vi "ID Finder.vi"(0 "cluster":T3 {"data[0]"."payload" format="%x"; "data[0]"."timestamp" format="%<%.7X\n%x>T"; "data[0]"."type" items=["CAN Data"=0, "CAN Remote"=1, "CAN Bus Error"=2, "CAN 2.0 Data"=8, "CAN FD Data"=16, "CAN FD+BRS Data"=24, "J1939 Data"=192, "Delay"=224, "Log Trigger"=225, "Start Trigger"=226]; "data[0]"."identifier" format="%x"; "data[1]"."payload" format="%x"; "data[1]"."timestamp" format="%<%.7X\n%x>T"; "data[1]"."type" items=["CAN Data"=0, "CAN Remote"=1, "CAN Bus Error"=2, "CAN 2.0 Data"=8, "CAN FD Data"=16, "CAN FD+BRS Data"=24, "J1939 Data"=192, "Delay"=224, "Log Trigger"=225, "Start Trigger"=226]; "data[1]"."identifier" format="%x"; "data[2]"."payload" format="%x"; "data[2]"."timestamp" format="%<%.7X\n%x>T"; "data[2]"."type" items=["CAN Data"=0, "CAN Remote"=1, "CAN Bus Error"=2, "CAN 2.0 Data"=8, "CAN FD Data"=16, "CAN FD+BRS Data"=24, "J1939 Data"=192, "Delay"=224, "Log Trigger"=225, "Start Trigger"=226]; "data[2]"."identifier" format="%x"; "data[3]"."payload" format="%x"; "data[3]"."timestamp" format="%<%.7X\n%x>T"; "data[3]"."type" items=["CAN Data"=0, "CAN Remote"=1, "CAN Bus Error"=2, "CAN 2.0 Data"=8, "CAN FD Data"=16, "CAN FD+BRS Data"=24, "J1939 Data"=192, "Delay"=224, "Log Trigger"=225, "Start Trigger"=226]; "data[3]"."identifier" format="%x"; "data[4]"."payload" format="%x"; "data[4]"."timestamp" format="%<%.7X\n%x>T"; "data[4]"."type" items=["CAN Data"=0, "CAN Remote"=1, "CAN Bus Error"=2, "CAN 2.0 Data"=8, "CAN FD Data"=16, "CAN FD+BRS Data"=24, "J1939 Data"=192, "Delay"=224, "Log Trigger"=225, "Start Trigger"=226]; "data[4]"."identifier" format="%x"; "data[5]"."payload" format="%x"; "data[5]"."timestamp" format="%<%.7X\n%x>T"; "data[5]"."type" items=["CAN Data"=0, "CAN Remote"=1, "CAN Bus Error"=2, "CAN 2.0 Data"=8, "CAN FD Data"=16, "CAN FD+BRS Data"=24, "J1939 Data"=192, "Delay"=224, "Log Trigger"=225, "Start Trigger"=226]; "data[5]"."identifier" format="%x"; "data[6]"."payload" format="%x"; "data[6]"."timestamp" format="%<%.7X\n%x>T"; "data[6]"."type" items=["CAN Data"=0, "CAN Remote"=1, "CAN Bus Error"=2, "CAN 2.0 Data"=8, "CAN FD Data"=16, "CAN FD+BRS Data"=24, "J1939 Data"=192, "Delay"=224, "Log Trigger"=225, "Start Trigger"=226]; "data[6]"."identifier" format="%x"; "data[7]"."payload" format="%x"; "data[7]"."timestamp" format="%<%.7X\n%x>T"; "data[7]"."type" items=["CAN Data"=0, "CAN Remote"=1, "CAN Bus Error"=2, "CAN 2.0 Data"=8, "CAN FD Data"=16, "CAN FD+BRS Data"=24, "J1939 Data"=192, "Delay"=224, "Log Trigger"=225, "Start Trigger"=226]; "data[7]"."identifier" format="%x"; "data[8]"."payload" format="%x"; "data[8]"."timestamp" format="%<%.7X\n%x>T"; "data[8]"."type" items=["CAN Data"=0, "CAN Remote"=1, "CAN Bus Error"=2, "CAN 2.0 Data"=8, "CAN FD Data"=16, "CAN FD+BRS Data"=24, "J1939 Data"=192, "Delay"=224, "Log Trigger"=225, "Start Trigger"=226]; "data[8]"."identifier" format="%x"}, 1 "ID ESPERADO STRING":string) -> (2 "Identifier":u32 format="%x", 3 "Data Type":T1 items=["CAN Data"=0, "CAN Remote"=1, "CAN Bus Error"=2, "CAN 2.0 Data"=8, "CAN FD Data"=16, "CAN FD+BRS Data"=24, "J1939 Data"=192, "Delay"=224, "Log Trigger"=225, "Start Trigger"=226], 4 "Timestamp":timestamp, 5 "Payload":u8[](array[numeric]) format="%x", 6 "ID String":string, 7 "Data String":string)   [LabVIEW 2023]
uses:
  <vilib>/xnet/xnet.llb/XNET Frame CAN.ctl
  <vilib>/xnet/xnet.llb/XNET Frame Type CAN.ctl
  C:/Elatch-Bench-Test/VIs 64 bits/Users/k90011005/Desktop/Practicas/C#/String-Hexa/bin/Debug/String-Hexa.dll
  VIs 64 bits/Users/k90011005/Desktop/Practicas/C#/String-Hexa/bin/Debug/String-Hexa.dll
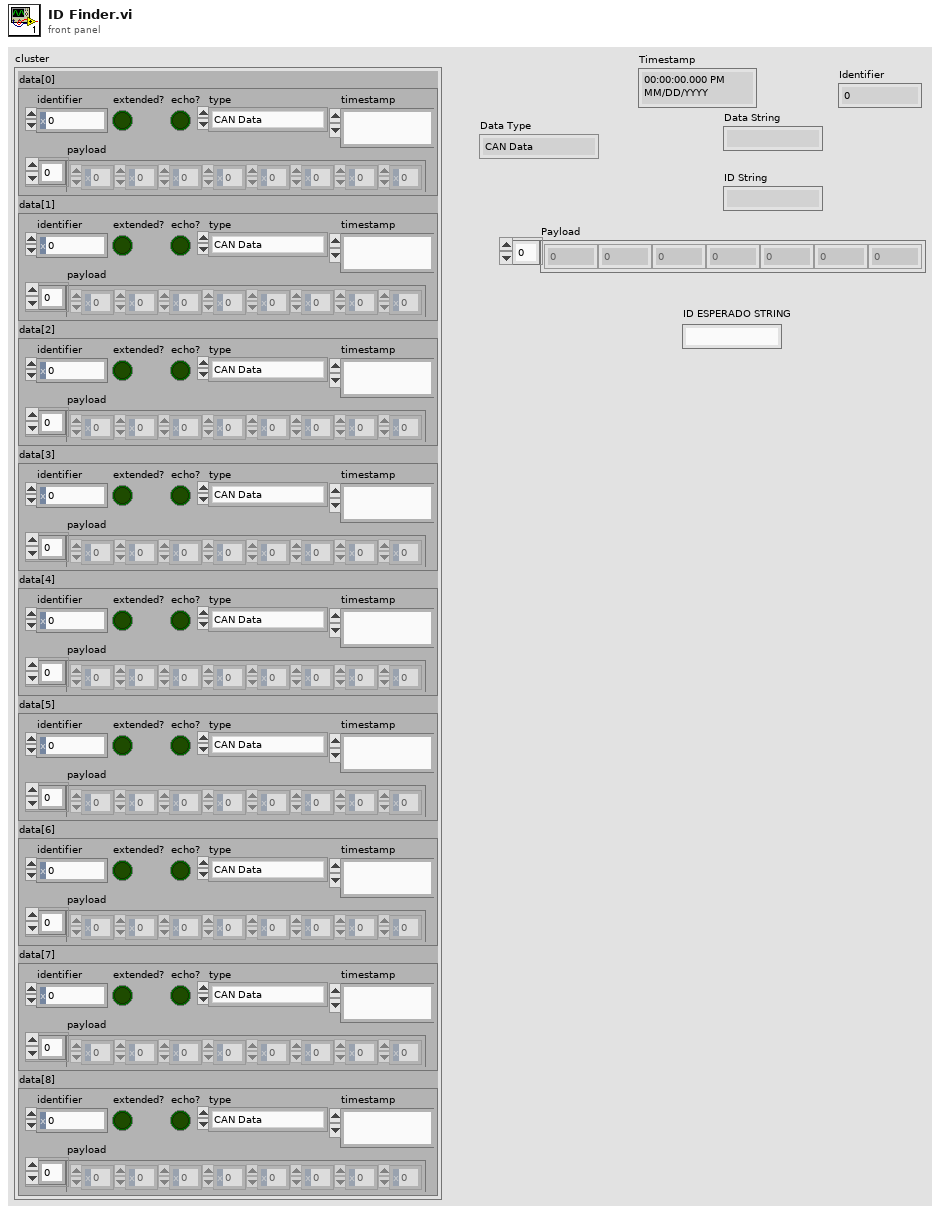
[diagram p1: front panel]
types:
  T1 = typedef "XNET Frame Type CAN.ctl" = u8
  T2 = typedef "XNET Frame CAN.ctl" = cluster{"timestamp":timestamp, "payload":u8[], "identifier":u32, "type":T1, "extended?":bool, "echo?":bool}
  T3 = cluster{"data[0]":T2, "data[1]":T2, "data[2]":T2, "data[3]":T2, "data[4]":T2, "data[5]":T2, "data[6]":T2, "data[7]":T2, "data[8]":T2}
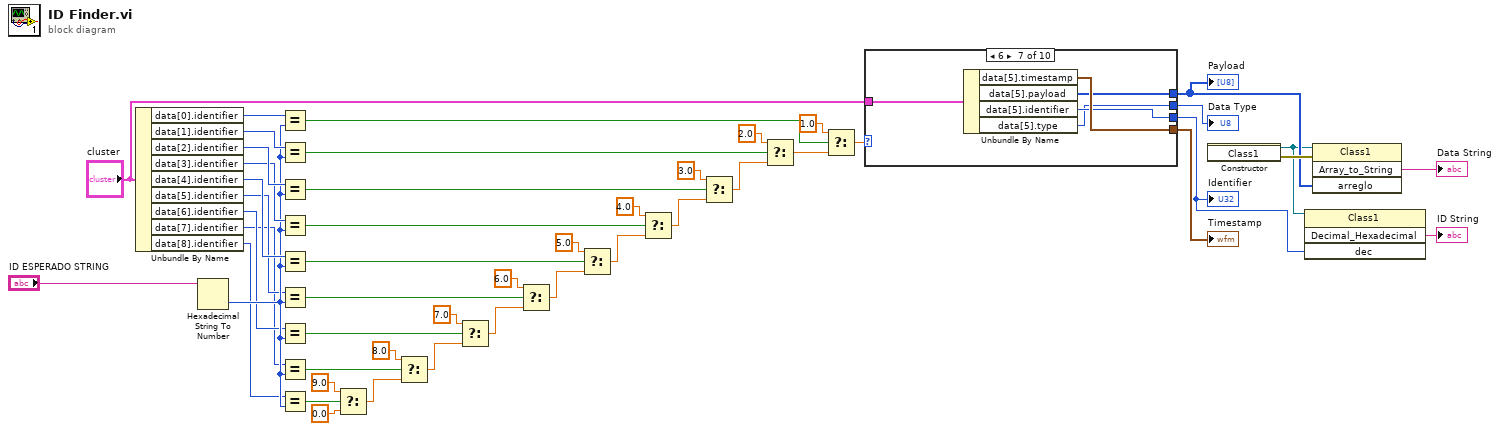
[diagram p0: block diagram]
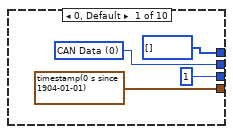
[diagram p2: hidden frame]
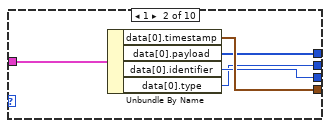
[diagram p3: hidden frame]
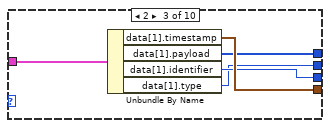
[diagram p4: hidden frame]
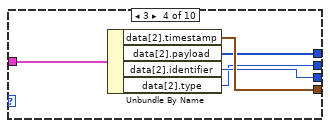
[diagram p5: hidden frame]
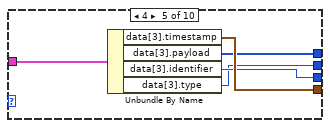
[diagram p6: hidden frame]
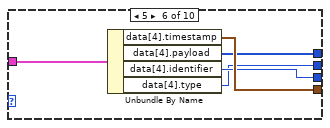
[diagram p7: hidden frame]
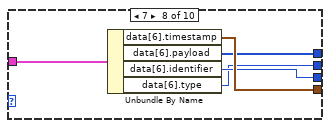
[diagram p8: hidden frame]
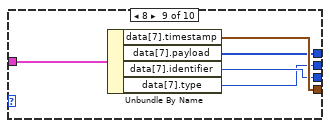
[diagram p9: hidden frame]
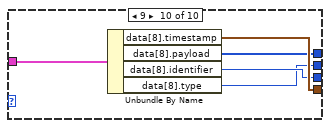
[diagram p10: hidden frame]
diagram:
  n1 = Unbundle By Name("cluster") -> ("data[0].identifier"=w48:u32, "data[1].identifier"=w43:u32, "data[2].identifier"=w42:u32, "data[3].identifier"=w41:u32, "data[4].identifier"=w40:u32, "data[5].identifier"=w9:u32, "data[6].identifier"=w8:u32, "data[7].identifier"=w7:u32, "data[8].identifier"=w6:u32)
  n2 = Hexadecimal String To Number(string="ID ESPERADO STRING") -> (number=w18:u32)  [unwired: 2 in, 1 out]
  n3 = Equal?(x=w48, y=w18) -> (x = y?=w47:bool)
  n4 = Equal?(x=w43, y=w18) -> (x = y?=w35:bool)
  n5 = Equal?(x=w42, y=w18) -> (x = y?=w34:bool)
  n6 = Equal?(x=w41, y=w18) -> (x = y?=w33:bool)
  n7 = Equal?(x=w40, y=w18) -> (x = y?=w32:bool)
  n8 = Equal?(x=w9, y=w18) -> (x = y?=w17:bool)
  n9 = Equal?(x=w8, y=w18) -> (x = y?=w16:bool)
  n10 = Equal?(x=w7, y=w18) -> (x = y?=w15:bool)
  n11 = Equal?(x=w6, y=w18) -> (x = y?=w14:bool)
  n12 = Select(t=9.0, s=w14, f=0.0) -> (s? t:f=w10:dbl)
  n13 = Select(t=8.0, s=w15, f=w10) -> (s? t:f=w11:dbl)
  n14 = Select(t=7.0, s=w16, f=w11) -> (s? t:f=w12:dbl)
  n15 = Select(t=6.0, s=w17, f=w12) -> (s? t:f=w13:dbl)
  n16 = Select(t=5.0, s=w32, f=w13) -> (s? t:f=w36:dbl)
  n17 = Select(t=4.0, s=w33, f=w36) -> (s? t:f=w37:dbl)
  n18 = Select(t=3.0, s=w34, f=w37) -> (s? t:f=w38:dbl)
  n19 = Select(t=2.0, s=w35, f=w38) -> (s? t:f=w39:dbl)
  n20 = Select(t=1.0, s=w47, f=w39) -> (s? t:f=w45:dbl)
  n21 = case shown="6" w45 {
    tunnel: "cluster" -> [_ w57 w62 w67 w72 w77 w82 w87 w88 w93]
    tunnel: [timestamp(0 s since 1904-01-01) ("timestamp") w56 w61 w66 w71 w76 w81 w86 w92 w97] -> w27
    tunnel: [u8[] [] ("payload") w55 w60 w65 w70 w75 w80 w85 w91 w94] -> w24
    tunnel: [u32 1 ("identifier") w54 w59 w64 w69 w74 w79 w84 w90 w96] -> w22
    tunnel: [w49 w53 w58 w63 w68 w73 w78 w83 w89 w95] -> w26
    frame 0, Default {
      w49 = T1 0 items=["CAN Data"=0, "CAN Remote"=1, "CAN Bus Error"=2, "CAN 2.0 Data"=8, "CAN FD Data"=16, "CAN FD+BRS Data"=24, "J1939 Data"=192, "Delay"=224, "Log Trigger"=225, "Start Trigger"=226] ("type")
    }
    frame 1 {
      n22 = Unbundle By Name(w57) -> ("data[0].timestamp"=w56:timestamp, "data[0].payload"=w55:u8[], "data[0].identifier"=w54:u32, "data[0].type"=w53:T1)
    }
    frame 2 {
      n23 = Unbundle By Name(w62) -> ("data[1].timestamp"=w61:timestamp, "data[1].payload"=w60:u8[], "data[1].identifier"=w59:u32, "data[1].type"=w58:T1)
    }
    frame 3 {
      n24 = Unbundle By Name(w67) -> ("data[2].timestamp"=w66:timestamp, "data[2].payload"=w65:u8[], "data[2].identifier"=w64:u32, "data[2].type"=w63:T1)
    }
    frame 4 {
      n25 = Unbundle By Name(w72) -> ("data[3].timestamp"=w71:timestamp, "data[3].payload"=w70:u8[], "data[3].identifier"=w69:u32, "data[3].type"=w68:T1)
    }
    frame 5 {
      n26 = Unbundle By Name(w77) -> ("data[4].timestamp"=w76:timestamp, "data[4].payload"=w75:u8[], "data[4].identifier"=w74:u32, "data[4].type"=w73:T1)
    }
    frame 6 {
      n27 = Unbundle By Name(w82) -> ("data[5].timestamp"=w81:timestamp, "data[5].payload"=w80:u8[], "data[5].identifier"=w79:u32, "data[5].type"=w78:T1)
    }
    frame 7 {
      n28 = Unbundle By Name(w87) -> ("data[6].timestamp"=w86:timestamp, "data[6].payload"=w85:u8[], "data[6].identifier"=w84:u32, "data[6].type"=w83:T1)
    }
    frame 8 {
      n29 = Unbundle By Name(w88) -> ("data[7].timestamp"=w92:timestamp, "data[7].payload"=w91:u8[], "data[7].identifier"=w90:u32, "data[7].type"=w89:T1)
    }
    frame 9 {
      n30 = Unbundle By Name(w93) -> ("data[8].timestamp"=w97:timestamp, "data[8].payload"=w94:u8[], "data[8].identifier"=w96:u32, "data[8].type"=w95:T1)
    }
  }
  "Timestamp" <- w27
  "Payload" <- w24
  "Identifier" <- w22
  "Data Type" <- w26
  n31 = constructor class="Class1"() -> (reference out=w21:refnum<k24>, error out=w25:errorcluster)  [unwired: 3 in, 1 out]
  n32 = invoke class="Class1" method="Decimal_Hexadecimal"(reference=w21, "dec"=w22) -> ("Decimal_Hexadecimal"=→"ID String":string)  [unwired: 2 in, 3 out]
  n33 = invoke class="Class1" method="Array_to_String"(reference=w21, error in=w25, "arreglo"=w24) -> ("Array_to_String"=→"Data String":string)  [unwired: 1 in, 3 out]
